vi "Data Read.vi"(6 "Append Index":i32 min=-1, 8 "error in (no error)":errorcluster, 11 "path":path) -> (0 "error out":errorcluster, 1 "Notes":string, 2 "Data (Dictionary)":T1[](array[typedef]), 3 "path out":path)   [LabVIEW 2016, in "LV-Data.lvclass"]
uses:
  LV-Data.lvclass
  Typedefs/Operation--enum.ctl
  Typedefs/File Type--enum.ctl
  Typedefs/Dictionary--cluster.ctl
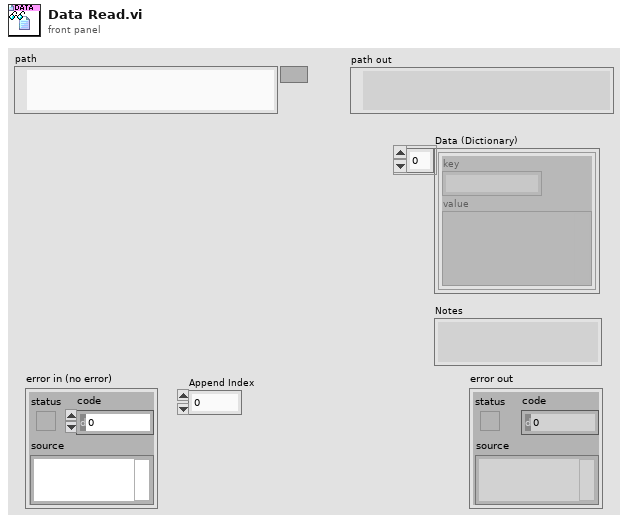
[diagram p1: front panel]
types:
  T1 = typedef "LV-Data.lvclass/Dictionary--cluster.ctl" = cluster{"key":string, "value":variant}
  T2 = typedef "LV-Data.lvclass/Operation--enum.ctl" = enum16{"Read", "Write", "Write + Append"}
  T3 = typedef "LV-Data.lvclass/File Type--enum.ctl" = enum16{"DAT", "ITX", "TDMS", "VI"}
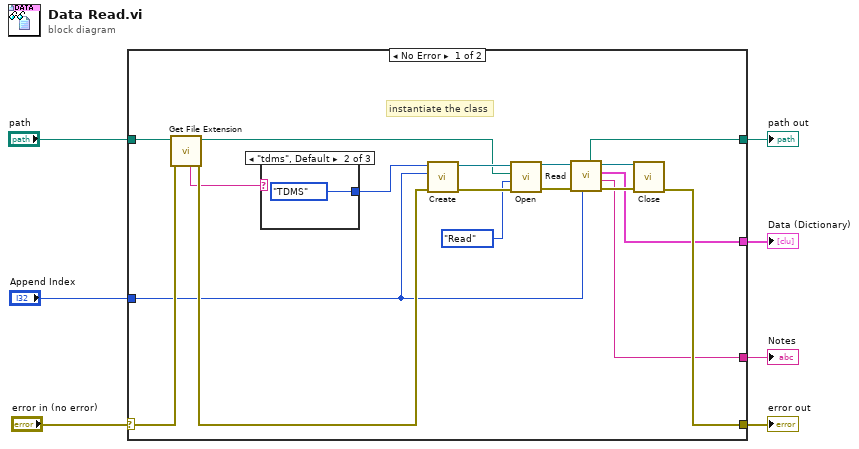
[diagram p0: block diagram]
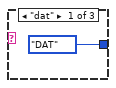
[diagram p2: hidden frame]
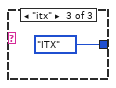
[diagram p3: hidden frame]
diagram:
  n1 = case shown="No Error" "error in (no error)" {
    selector: "error in (no error)" -> [w15 w30]
    tunnel: [w19 w30] -> w6
    tunnel: [w18 w29] -> w5
    tunnel: "path" -> [w13 w29]
    tunnel: [w17 _] -> w2
    tunnel: [w16 _] -> w3
    tunnel: "Append Index" -> [w10 _]
    frame No Error {
      # "instantiate the class"
      n2 = call <vilib>:"Get File Extension.vi"("error in (no error)"=w15, "file"=w13) -> ("error out"=w14:errorcluster, "dup file"=w9:path, "unmodified file extension"=w12:string)  [unwired: 5 in, 2 out]
      n3 = case shown="\"tdms\", Default" w12 {
        tunnel: [File_Type--enum."DAT" ("File Type") File_Type--enum."TDMS" ("File Type") File_Type--enum."ITX" ("File Type")] -> w11
        frame "dat" {
        }
        frame "tdms", Default {
        }
        frame "itx" {
        }
      }
      n4 = call "Create.vi"("error in (no error)"=w14, "Append Index (-1)"=w10, "File Type"=w11) -> ("error out"=w24:errorcluster, "Data out"=w25:refnum<class "LV-Data.lvclass">)  [unwired: 7 in]
      n5 = call-dynamic "Open.vi"("error in (no error)"=w24, "Operation"=Operation--enum."Read", "Path"=w9, "Data in"=w25) -> ("error out"=w22:errorcluster, "Data out"=w23:refnum<class "LV-Data.lvclass">)  [unwired: 6 in]
      n6 = call-dynamic "Read.vi"("Append Index"=w10, "error in (no error)"=w22, "Data Save in"=w23) -> ("error out"=w21:errorcluster, "Notes"=w16:string, "Data (Dictionary)"=w17:T1[], "Data Save out"=w20:refnum<class "LV-Data.lvclass">, "Path out"=w18:path)  [unwired: 4 in]
      n7 = call-dynamic "Close.vi"("error in (no error)"=w21, "Data in"=w20) -> ("error out"=w19:errorcluster)  [unwired: 8 in, 1 out]
    }
    frame Error {
    }
  }
  "error out" <- w6
  "path out" <- w5
  "Data (Dictionary)" <- w2
  "Notes" <- w3
